vi "Get DDG Insertion Delay.vi"(11 "piState":i32) -> (2 "function return":u32, 3 "piState out":i32)   [LabVIEW 2018, in "AndorSDK.lvlib"]
doc: "EXPNETTYPE unsigned int WINAPI GetDDGInsertionDelay(int * piState);"
uses:
  AndorSDK.lvlib
  ATMCD32D.dll
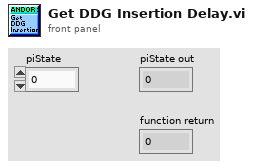
[diagram p1: front panel]
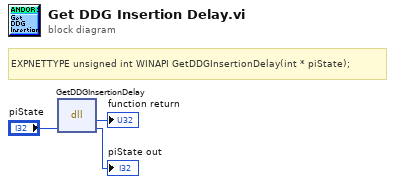
[diagram p0: block diagram]
diagram:
  # "EXPNETTYPE unsigned int WINAPI GetDDGInsertionDelay(int * piState);"
  n1 = dll-call lib="PTH2babs E\nPersönliches02 - Arbeit03-HiwijobsLabviewCodelibANDOR\tAndor SDK\nATMCD32D.*" fn="GetDDGInsertionDelay"("piState"="piState") -> (→"function return":u32, "piState"=→"piState out":i32)  [unwired: 3 in, 2 out]
